vi "OA Get User Mode Names.vi"(8 "error in (no error)":errorcluster, 11 "pcListOfModes":string) -> (0 "error out":errorcluster, 2 "function return":u32, 3 "pcListOfModes out":string)   [LabVIEW 2014, in "atmcd32d.lvlib"]
doc: "unsigned int WINAPI OA_GetUserModeNames(char * pcListOfModes);"
uses:
  atmcd32d.lvlib
  atmcd32d.dll
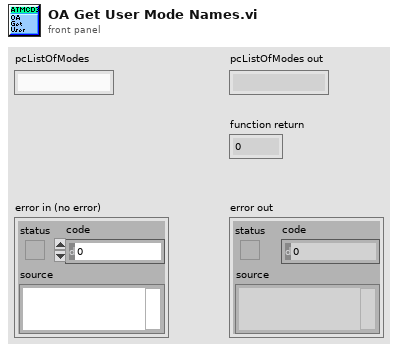
[diagram p1: front panel]
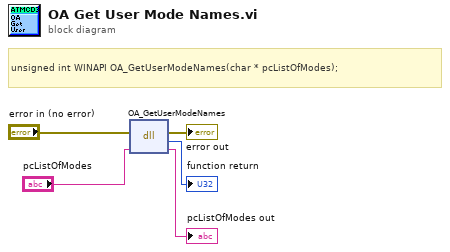
[diagram p0: block diagram]
diagram:
  # "unsigned int WINAPI OA_GetUserModeNames(char * pcListOfModes);"
  n1 = dll-call lib="C:/Users/Bakir/Documents/Lambda2-Testing/lib/Andorlib/atmcd32d.*" fn="OA_GetUserModeNames"(error in="error in (no error)", "pcListOfModes"="pcListOfModes") -> (error out=→"error out":errorcluster, →"function return":u32, "pcListOfModes"=→"pcListOfModes out":string)  [unwired: 2 in, 1 out]
